vi "USRP_singlecarrierTDMUSRP1_conf.vi"() -> ()   [LabVIEW 2021]
uses:
  <vilib>/addons/Modulation/Analog/controls/Complex Data Waveform.ctl
  <vilib>/Analysis/coordinate.llb/Angle Units.ctl
  <vilib>/Analysis/coordinate.llb/Angle Range (Degree).ctl
  <vilib>/Analysis/coordinate.llb/Wrap Angle (scalar).vi
  system stop.vi
  <vilib>/measure/matone.llb/Extract Single Tone Information 1 Chan (CDB).vi
  <instrlib>/niUSRP/niUSRP Fetch Rx Data (CDB Cluster).vi
  <instrlib>/niUSRP/niUSRP Write Tx Data (CDB Cluster).vi
  <vilib>/addons/Modulation/niAMT.lvlib
  <vilib>/measure/NI_MAPro.lvlib
  <vilib>/Analysis/NI_AAL_Angle.lvlib
panel:
  in  "Tab Control":T1(tab)
  in  "IQ rate Tx":dbl=400000.0 format="%#_6p"
  in  "Tx Gain":dbl format="%#_6f"
  in  "Tx IP":refnum<k15>="192.168.10.2"
  out "coerced IQ rate Tx":dbl=100000.0 format="%#_6p"
  out "coerced carrier frequency Tx":dbl=100000.0 format="%#_6p"
  in  "Rx IP":refnum<k15>="192.168.10.2"
  in  "Rx gain":dbl format="%#_6f"
  in  "Frequency":dbl=10000.0 format="%#_13g"
  in  "Duration":dbl=0.01 format="%#_13g"
  out "coerced IQ rate Rx":dbl=100000.0 format="%#_6p"
  out "coerced carrier frequency Rx":dbl=100000.0 format="%#_6p"
  in  "number of samples":i64=4000
  in  "carrier frequency":dbl=2400000000.0 format="%#_6p"
  in  "Phase in deg":dbl
  out "Counter":dbl
  out "Waveform Graph":dbl[](graph)
  out "Boolean":bool
  out "detected frequency":dbl format="%.2p"
  out "detected Amplitude":dbl format="%.2p"
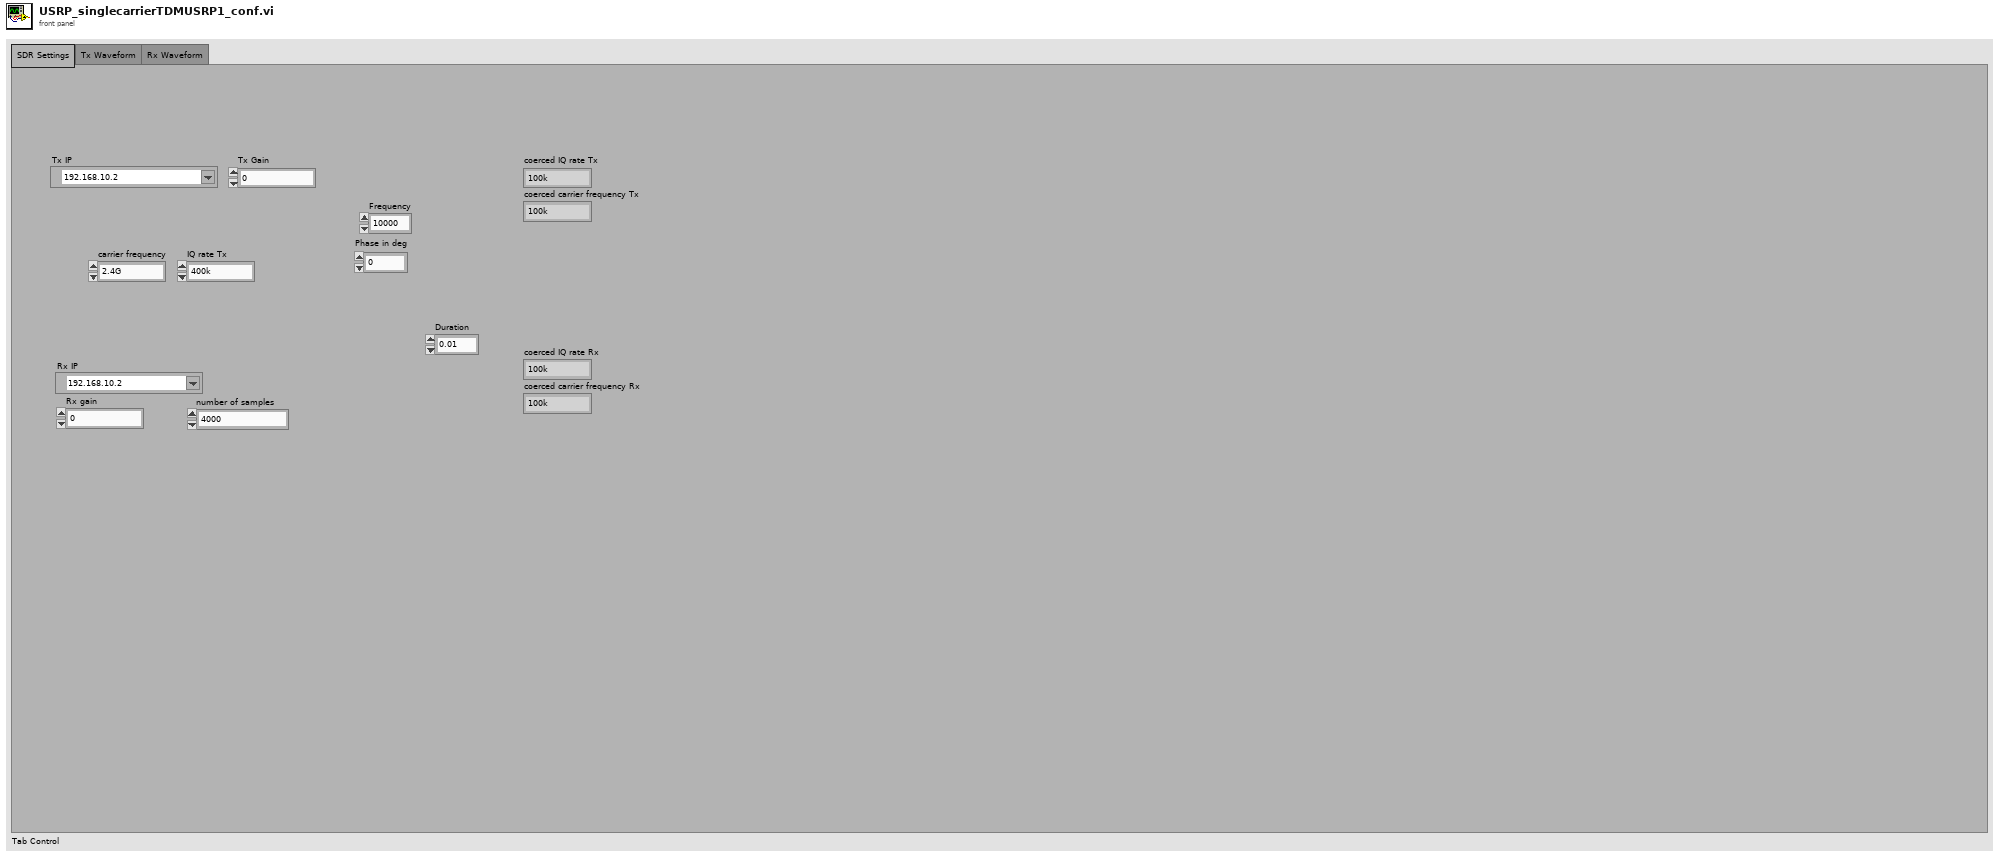
[diagram p1: front panel]
types:
  T1 = enum32{"SDR Settings", "Tx Waveform", "Rx Waveform"}
  T2 = typedef "niAMT.lvlib/Complex Data Waveform.ctl" = cluster{"t0":dbl, "dt":dbl, "Y":cdb[]}
  T3 = typedef "NI_AAL_Angle.lvlib/Angle Range (Degree).ctl" = u16
  T4 = typedef "NI_AAL_Angle.lvlib/Angle Units.ctl" = i32
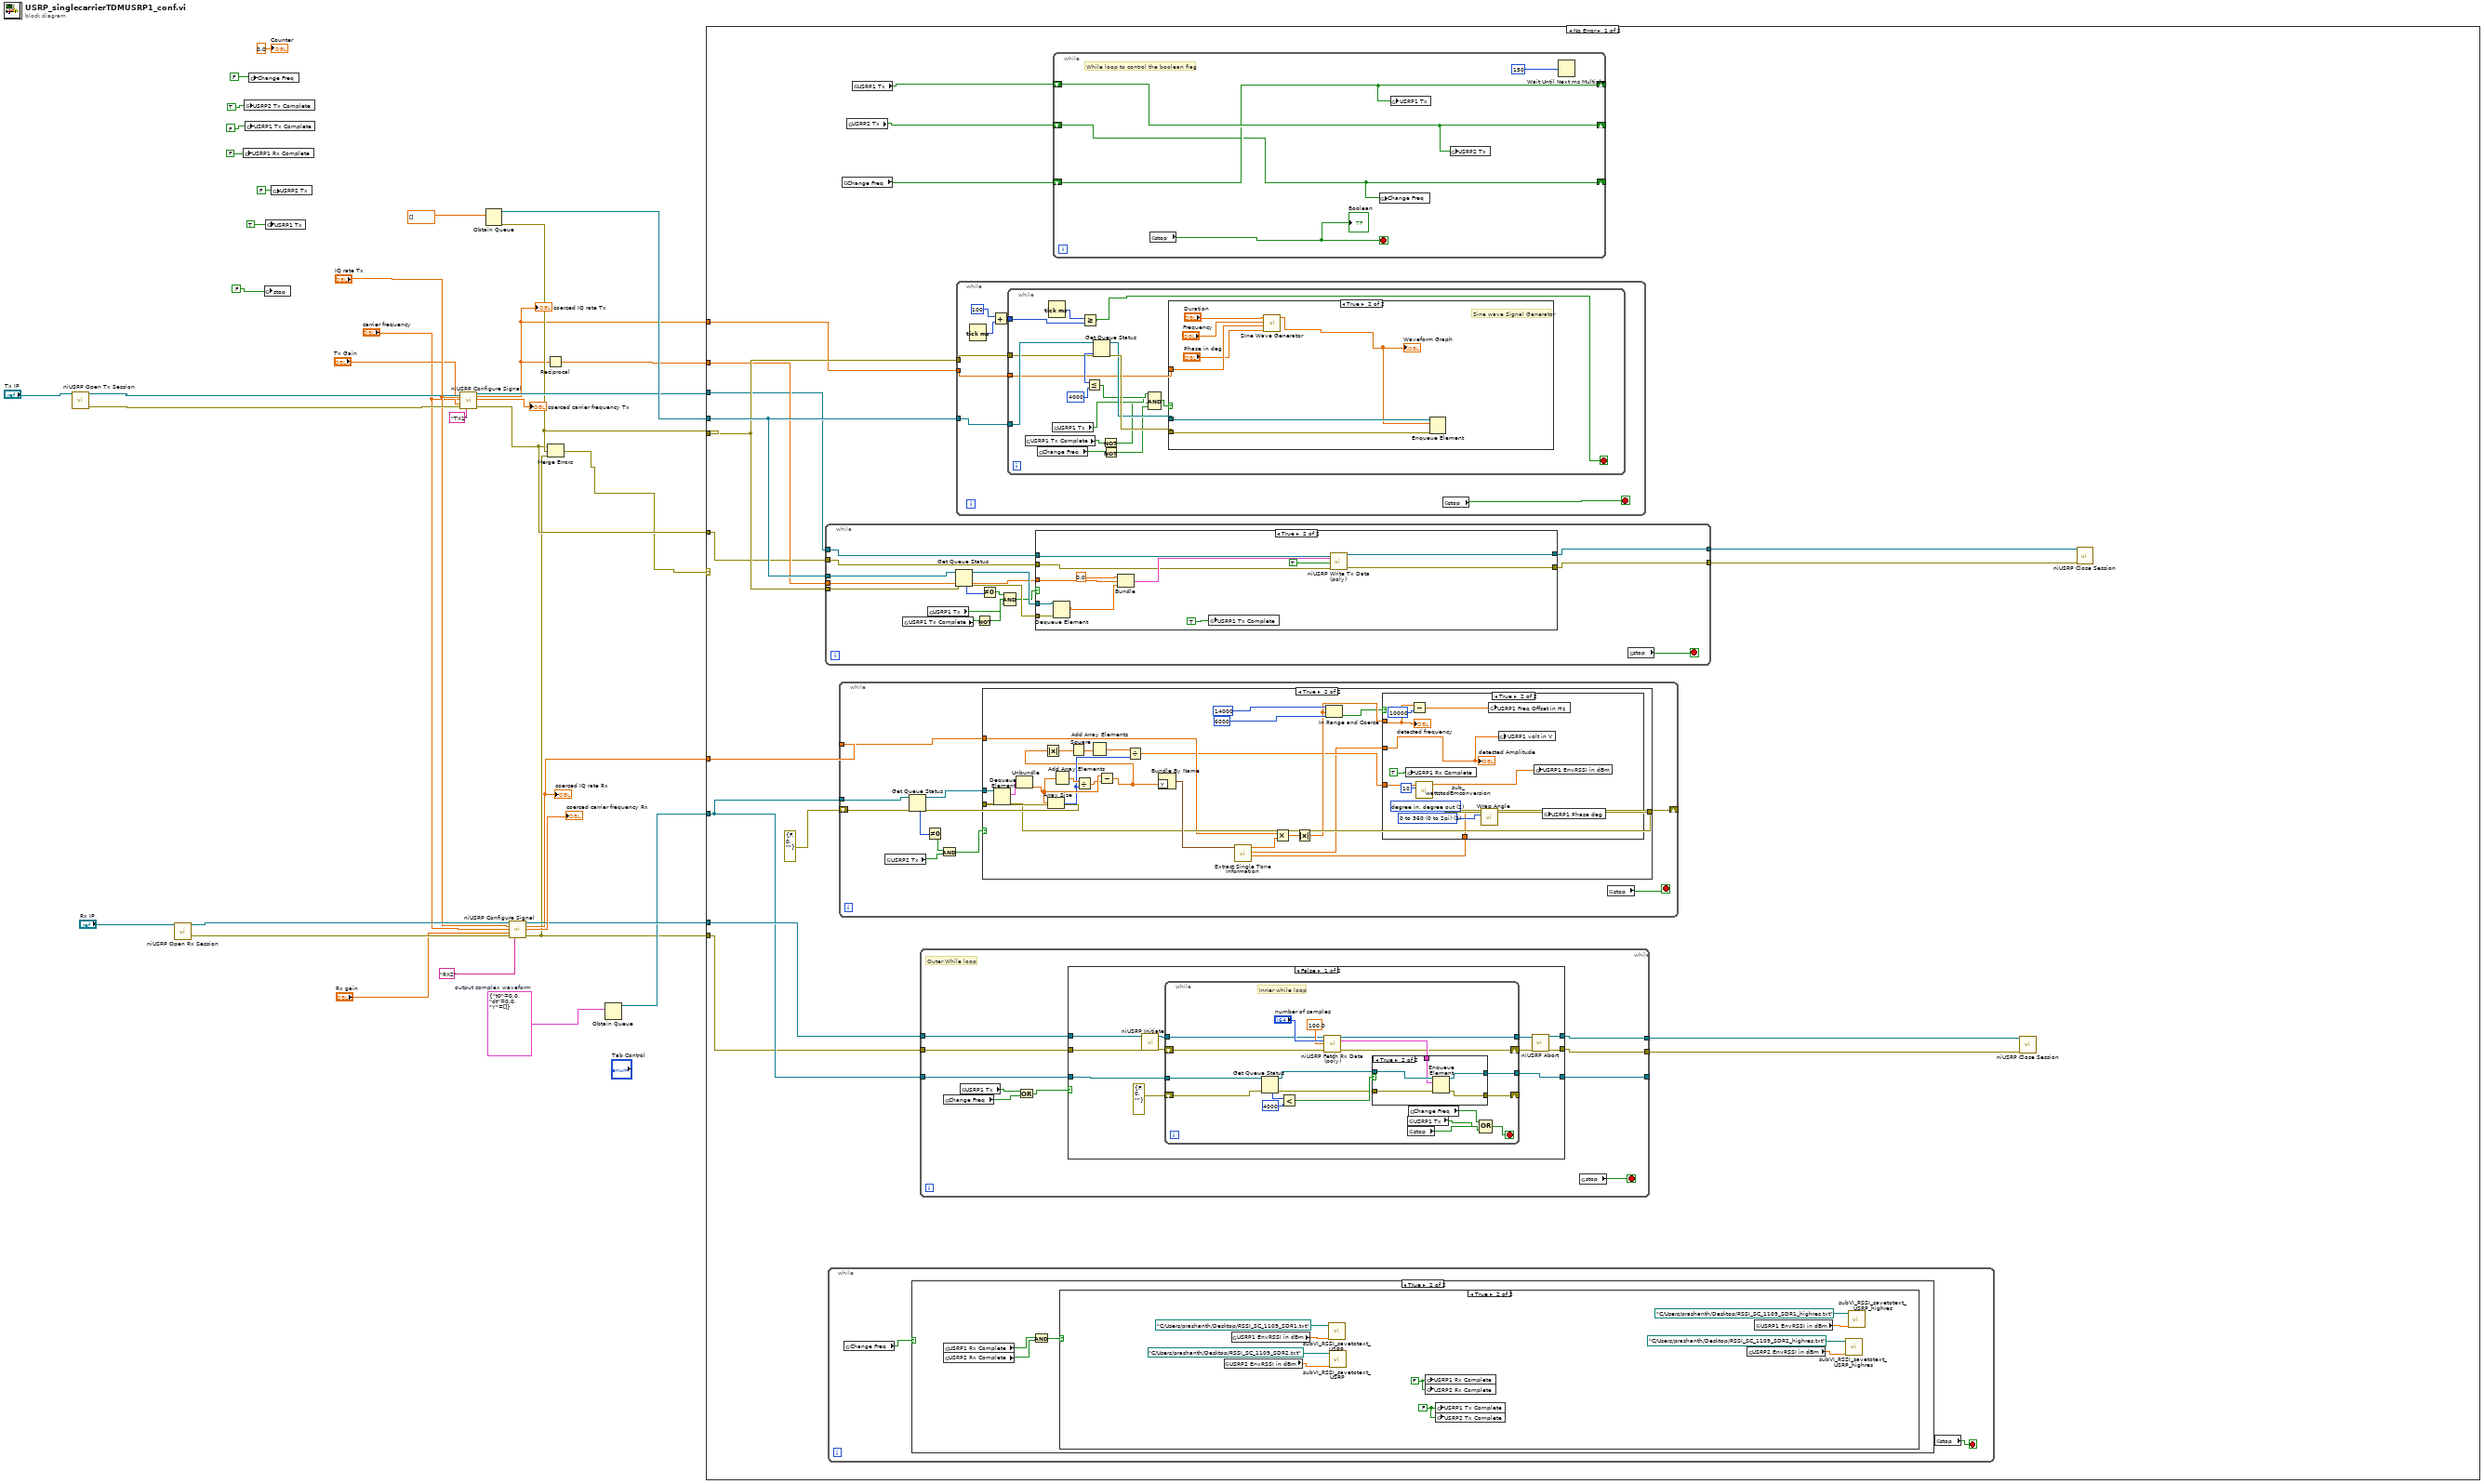
[diagram p0: block diagram]
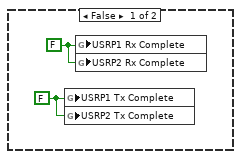
[diagram p3: hidden frame]
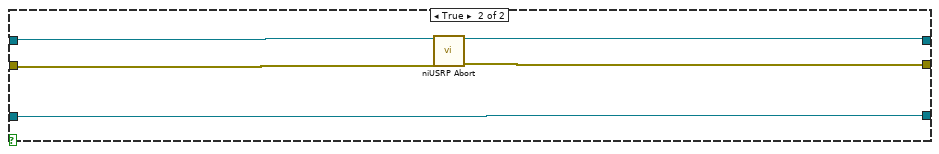
[diagram p6: hidden frame]
diagram:
  w9 = T2 {"t0"=0.0, "dt"=0.0, "Y"=[]}  # output complex waveform
  n1 = call <instrlib>:"niUSRP Open Tx Session.vi"("device names"="Tx IP") -> ("session handle out"=w34:refnum<k15>, "error out"=w33:errorcluster)  [unwired: 13 in]
  n2 = call <instrlib>:"niUSRP Open Rx Session.vi"("device names"="Rx IP") -> ("session handle out"=w31:refnum<k15>, "error out"=w30:errorcluster)  [unwired: 13 in]
  n3 = global write "system stop.vi" "USRP1 Rx Complete"(FALSE) -> ()
  n4 = global write "system stop.vi" "USRP2 Tx Complete"(TRUE) -> ()
  n5 = global write "system stop.vi" "USRP1 Tx Complete"(FALSE) -> ()
  n6 = global write "system stop.vi" "Change Freq"(FALSE) -> ()
  n7 = global write "system stop.vi" "stop"(FALSE) -> ()
  n8 = global write "system stop.vi" "USRP1 Tx"(TRUE) -> ()
  n9 = global write "system stop.vi" "USRP2 Tx"(FALSE) -> ()
  n10 = call <instrlib>:"niUSRP Configure Signal.vi"("session handle"=w34, "IQ rate"="IQ rate Tx", "carrier frequency"="carrier frequency", "gain"="Tx Gain", "error in (no error)"=w33, "active antenna"="TX1") -> ("session handle out"=w16:refnum<k15>, "coerced IQ rate"=w13:dbl, "coerced carrier frequency"=→"coerced carrier frequency Tx":dbl, "error out"=w12:errorcluster)  [unwired: 5 in, 1 out]
  "coerced IQ rate Tx" <- w13
  n11 = Obtain Queue(element data type=dbl[] []) -> (queue out=w17:refnum<queue>, error out=w14:errorcluster)  [unwired: 4 in, 1 out]
  n12 = call <instrlib>:"niUSRP Configure Signal.vi"("session handle"=w31, "IQ rate"="IQ rate Tx", "carrier frequency"="carrier frequency", "gain"="Rx gain", "error in (no error)"=w30, "active antenna"="RX2") -> ("session handle out"=w10:refnum<k15>, "coerced IQ rate"=w7:dbl, "coerced carrier frequency"=→"coerced carrier frequency Rx":dbl, "error out"=w6:errorcluster)  [unwired: 5 in, 1 out]
  "coerced IQ rate Rx" <- w7
  n13 = Reciprocal(x=w13) -> (1/x=w15:dbl)
  n14 = Merge Errors(w12, w14, w6) -> (w4:errorcluster)
  n15 = Obtain Queue(element data type=w9) -> (queue out=w8:refnum<queue>)  [unwired: 4 in, 2 out]
  n16 = case shown="No Error" w4 {
    tunnel: w14 -> [w52 _]
    tunnel: w17 -> [w53 _]
    tunnel: w16 -> [w50 _]
    tunnel: w15 -> [w51 _]
    tunnel: w13 -> [w49 _]
    tunnel: w12 -> [w48 _]
    tunnel: w10 -> [w46 _]
    tunnel: w8 -> [w45 _]
    tunnel: w7 -> [w44 _]
    tunnel: w6 -> [w43 _]
    frame No Error {
      n17 = while {
        tunnel: w52 -> [w219]
        tunnel: w51 -> [w218]
        tunnel: w50 -> [w215]
        tunnel: w48 -> [w214]
        tunnel: [w210] -> w39
        tunnel: [w209] -> w38
        tunnel: w53 -> [w222]
        stop <- w216 stop-if-true
        n18 = global read "system stop.vi" "USRP1 Tx Complete"() -> (w211:bool)
        n19 = global read "system stop.vi" "USRP1 Tx"() -> (w207:bool)
        n20 = Get Queue Status(queue=w222, error in (no error)=w219) -> (queue out=w221:refnum<queue>, error out=w220:errorcluster, # elements in queue=w217:i32)  [unwired: 1 in, 5 out]
        n21 = Not(x=w211) -> (.not. x?=w212:bool)
        n22 = Not Equal To 0?(x=w217) -> (x != 0?=w213:bool)
        n23 = Compound Arithmetic op=AND(w213, w212, w207) -> (w208:bool)
        n24 = case shown="True" w208 {
          tunnel: w221 -> [_ w236]
          tunnel: w220 -> [_ w235]
          tunnel: w218 -> [_ w234]
          tunnel: w215 -> [w224 w227]
          tunnel: w214 -> [w223 w226]
          tunnel: [w224 w230] -> w210
          tunnel: [w223 w228] -> w209
          frame False {
          }
          frame True {
            n25 = Dequeue Element(queue=w236, error in (no error)=w235) -> (element=w225:dbl[])  [unwired: 1 in, 3 out]
            n26 = Bundle(0.0, w234, w225) -> (w233:cluster{dbl, dbl, dbl[]})  [unwired: 1 in]
            n27 = global write "system stop.vi" "USRP1 Tx Complete"(TRUE) -> ()
            n28 = call-poly <instrlib>:"niUSRP Write Tx Data (poly).vi"("session handle"=w227, "data"=w233, "end of data?"=TRUE, "error in (no error)"=w226) -> ("session handle out"=w230:refnum<k15>, "error out"=w228:errorcluster)  [unwired: 10 in]
          }
        }
        n29 = global read "system stop.vi" "stop"() -> (w216:bool)
      }
      n30 = while {
        stop <- w54 stop-if-true
        n31 = global read "system stop.vi" "Change Freq"() -> (w55:bool)
        n32 = case shown="True" w55 {
          frame False {
          }
          frame True {
            n33 = global read "system stop.vi" "USRP1 Rx Complete"() -> (w58:bool)
            n34 = global read "system stop.vi" "USRP2 Rx Complete"() -> (w57:bool)
            n35 = And(x=w58, y=w57) -> (x .and. y?=w56:bool)
            n36 = case shown="True" w56 {
              frame False {
                w60 = FALSE
                w59 = FALSE
                n37 = global write "system stop.vi" "USRP1 Tx Complete"(w60) -> ()
                n38 = global write "system stop.vi" "USRP2 Tx Complete"(w60) -> ()
                n39 = global write "system stop.vi" "USRP1 Rx Complete"(w59) -> ()
                n40 = global write "system stop.vi" "USRP2 Rx Complete"(w59) -> ()
              }
              frame True {
                w70 = FALSE
                w69 = FALSE
                n41 = global read "system stop.vi" "USRP2 EnvRSSI in dBm"() -> (w61:dbl)
                n42 = global read "system stop.vi" "USRP1 EnvRSSI in dBm"() -> (w63:dbl)
                n43 = call "subVI_RSSI_savetotext_USRP.vi"("RSSI"=w63, "file path (dialog if empty)"=path "C:/Users/prashanth/Desktop/RSSI_SC_1109_SDR1.txt") -> ()  [unwired: 10 in]
                n44 = call "subVI_RSSI_savetotext_USRP.vi"("RSSI"=w61, "file path (dialog if empty)"=path "C:/Users/prashanth/Desktop/RSSI_SC_1109_SDR2.txt") -> ()  [unwired: 10 in]
                n45 = global write "system stop.vi" "USRP1 Rx Complete"(w69) -> ()
                n46 = global write "system stop.vi" "USRP2 Rx Complete"(w69) -> ()
                n47 = global write "system stop.vi" "USRP1 Tx Complete"(w70) -> ()
                n48 = global write "system stop.vi" "USRP2 Tx Complete"(w70) -> ()
                n49 = global read "system stop.vi" "USRP2 EnvRSSI in dBm"() -> (w67:dbl)
                n50 = global read "system stop.vi" "USRP1 EnvRSSI in dBm"() -> (w65:dbl)
                n51 = call "subVI_RSSI_savetotext_USRP_highres.vi"("RSSI"=w67, "file path (dialog if empty)"=path "C:/Users/prashanth/Desktop/RSSI_SC_1109_SDR2_highres.txt") -> ()  [unwired: 10 in]
                n52 = call "subVI_RSSI_savetotext_USRP_highres.vi"("RSSI"=w65, "file path (dialog if empty)"=path "C:/Users/prashanth/Desktop/RSSI_SC_1109_SDR1_highres.txt") -> ()  [unwired: 10 in]
              }
            }
          }
        }
        n53 = global read "system stop.vi" "stop"() -> (w54:bool)
      }
      n54 = while {
        tunnel: w45 -> [w167]
        shift-right: [w165] -> _
        shift-left: errorcluster {"status"=FALSE, "code"=0, "source"=""} ("error in (no error)") -> [w166]
        tunnel: w44 -> [w164]
        stop <- w163 stop-if-true
        n55 = global read "system stop.vi" "USRP2 Tx"() -> (w162:bool)
        n56 = Get Queue Status(queue=w167, error in (no error)=w166) -> (queue out=w169:refnum<queue>, error out=w168:errorcluster, # elements in queue=w170:i32)  [unwired: 1 in, 5 out]
        n57 = Not Equal To 0?(x=w170) -> (x != 0?=w161:bool)
        n58 = And(x=w161, y=w162) -> (x .and. y?=w160:bool)
        n59 = case shown="True" w160 {
          tunnel: w169 -> [_ w194]
          tunnel: w168 -> [w171 w193]
          tunnel: [w171 w187] -> w165
          tunnel: w164 -> [_ w185]
          frame False {
          }
          frame True {
            n60 = Dequeue Element(queue=w194, error in (no error)=w193) -> (element=w192:T2, error out=w187:errorcluster)  [unwired: 1 in, 2 out]
            n61 = Unbundle(w192) -> ("Y"=w182:cdb[])  [unwired: 2 out]
            n62 = Array Size(array=w182) -> (size(s)=w179:i32)
            n63 = Add Array Elements(numeric array=w182) -> (sum=w191:cdb)
            n64 = Divide(x=w191, y=w179) -> (x/y=w180:cdb)
            n65 = Subtract(x=w182, y=w180) -> (x-y=w174:cdb[])
            n66 = Absolute Value(x=w174) -> (abs(x)=w181:dbl[])
            n67 = Square(x=w181) -> (x^2=w178:dbl[])
            n68 = Add Array Elements(numeric array=w178) -> (sum=w177:dbl)
            n69 = Divide(x=w177, y=w179) -> (x/y=w176:dbl)
            n70 = Bundle By Name("Y"=w174) -> (w188:waveform(cdb))  [unwired: 1 in]
            n71 = call-poly <vilib>:"Extract Single Tone Information.vi"("time signal in"=w188) -> ("detected phase (deg)"=w175:dbl, "detected amplitude"=w173:dbl, "detected frequency"=w186:dbl)  [unwired: 5 in, 3 out]
            n72 = Multiply(x=w185, y=w186) -> (x*y=w184:dbl)
            n73 = Absolute Value(x=w184) -> (abs(x)=w183:dbl)
            n74 = In Range and Coerce(upper limit=14000, x=w183, lower limit=6000) -> (In Range?=w172:bool)  [unwired: 1 out]
            n75 = case shown="True" w172 {
              tunnel: w183 -> [_ w205]
              tunnel: w173 -> [_ w195]
              tunnel: w176 -> [_ w202]
              tunnel: w175 -> [_ w197]
              frame False {
              }
              frame True {
                w199 = T3 2 items=["none", "-180 to 180 (-pi to pi)", "0 to 360 (0 to 2pi)"] ("angle range")
                w200 = T4 2 items=["radian in, radian out", "radian in, degree out", "degree in, degree out", "degree in, radian out"] ("angle units")
                n76 = global write "system stop.vi" "USRP1 Rx Complete"(TRUE) -> ()
                n77 = Subtract(x=w205, y=10000) -> (x-y=w203:dbl)
                n78 = call "sub_wattstodBmconversion.vi"("Amp or Power"=10, "detected amplitude"=w202) -> ("Numeric"=w201:dbl)  [unwired: 9 in]
                n79 = call-poly <vilib>:"Wrap Angle.vi"("angle units"=w200, "angle range"=w199, "angle in"=w197) -> ("angle out"=w198:dbl)  [unwired: 7 in, 1 out]
                n80 = global write "system stop.vi" "USRP1 Freq Offset in Hz"(w203) -> ()
                n81 = global write "system stop.vi" "USRP1 volt in V"(w195) -> ()
                n82 = global write "system stop.vi" "USRP1 EnvRSSI in dBm"(w201) -> ()
                n83 = global write "system stop.vi" "USRP1 Phase deg"(w198) -> ()
                "detected frequency" <- w205
                "detected Amplitude" <- w195
              }
            }
          }
        }
        n84 = global read "system stop.vi" "stop"() -> (w163:bool)
      }
      n85 = global read "system stop.vi" "Change Freq"() -> (w41:bool)
      n86 = global read "system stop.vi" "USRP2 Tx"() -> (w40:bool)
      n87 = global read "system stop.vi" "USRP1 Tx"() -> (w42:bool)
      n88 = while {
        tunnel: w46 -> [w114]
        tunnel: w43 -> [w113]
        tunnel: [w108] -> w37
        tunnel: [w107] -> w36
        tunnel: w45 -> [w116]
        tunnel: [w112] -> _
        stop <- w115 stop-if-true
        # "Outer While loop"
        n89 = global read "system stop.vi" "Change Freq"() -> (w109:bool)
        n90 = global read "system stop.vi" "USRP1 Tx"() -> (w110:bool)
        n91 = Compound Arithmetic op=OR(w110, w109) -> (w111:bool)
        n92 = case shown="False" w111 {
          tunnel: w114 -> [w119 w159]
          tunnel: w116 -> [w127 w155]
          tunnel: w113 -> [w118 w157]
          tunnel: [w122 w158] -> w108
          tunnel: [w121 w156] -> w107
          tunnel: [w117 w155] -> w112
          frame False {
            n93 = call <instrlib>:"niUSRP Initiate.vi"("session handle"=w119, "error in (no error)"=w118) -> ("session handle out"=w125:refnum<k15>, "error out"=w124:errorcluster)  [unwired: 12 in]
            n94 = while {
              tunnel: w127 -> [w147]
              shift-right: [w131] -> w120
              shift-left: w124 -> [w133]
              shift-right: [w146] -> _
              shift-left: errorcluster {"status"=FALSE, "code"=0, "source"=""} ("error in (no error)") -> [w145]
              tunnel: w125 -> [w134]
              tunnel: [w132] -> w123
              tunnel: [w128] -> w117
              stop <- w137 stop-if-true
              # "Inner while loop"
              n95 = Get Queue Status(queue=w147, error in (no error)=w145) -> (queue out=w140:refnum<queue>, error out=w141:errorcluster, # elements in queue=w144:i32)  [unwired: 1 in, 5 out]
              n96 = Less?(x=w144, y=4000) -> (x < y?=w142:bool)
              n97 = call-poly <instrlib>:"niUSRP Fetch Rx Data (poly).vi"("session handle"=w134, "number of samples"="number of samples", "timeout"=100.0, "error in (no error)"=w133) -> ("session handle out"=w132:refnum<k15>, "data"=w138:cluster{"t0":dbl, "dt":dbl, "Y":cdb[]}, "error out"=w131:errorcluster)  [unwired: 8 in, 1 out]
              n98 = case shown="True" w142 {
                tunnel: w141 -> [w149 w154]
                tunnel: w140 -> [w148 w153]
                tunnel: w138 -> [_ w152]
                tunnel: [w149 w151] -> w146
                tunnel: [w148 w150] -> w128
                frame False {
                }
                frame True {
                  n99 = Enqueue Element(queue=w153, element=w152, error in (no error)=w154) -> (queue out=w150:refnum<queue>, error out=w151:errorcluster)  [unwired: 1 in, 1 out]
                }
              }
              n100 = global read "system stop.vi" "USRP1 Tx"() -> (w130:bool)
              n101 = global read "system stop.vi" "stop"() -> (w136:bool)
              n102 = global read "system stop.vi" "Change Freq"() -> (w129:bool)
              n103 = Compound Arithmetic op=OR(w129, w130, w136) -> (w137:bool)
            }
            n104 = call <instrlib>:"niUSRP Abort.vi"("session handle"=w123, "error in (no error)"=w120) -> ("session handle out"=w122:refnum<k15>, "error out"=w121:errorcluster)  [unwired: 12 in]
          }
          frame True {
            n105 = call <instrlib>:"niUSRP Abort.vi"("session handle"=w159, "error in (no error)"=w157) -> ("session handle out"=w158:refnum<k15>, "error out"=w156:errorcluster)  [unwired: 12 in]
          }
        }
        n106 = global read "system stop.vi" "stop"() -> (w115:bool)
      }
      n107 = while {
        tunnel: w52 -> [w81]
        tunnel: w49 -> [w80]
        tunnel: w53 -> [w82]
        stop <- w76 stop-if-true
        n108 = Tick Count (ms)() -> (millisecond timer value=w78:u32)
        n109 = Add(x=100, y=w78) -> (x+y=w77:u32)
        n110 = while {
          tunnel: w81 -> [w94]
          tunnel: w80 -> [w93]
          tunnel: w77 -> [w88]
          tunnel: w82 -> [w95]
          stop <- w84 stop-if-true
          n111 = global read "system stop.vi" "USRP1 Tx Complete"() -> (w86:bool)
          n112 = global read "system stop.vi" "Change Freq"() -> (w85:bool)
          n113 = Tick Count (ms)() -> (millisecond timer value=w89:u32)
          n114 = global read "system stop.vi" "USRP1 Tx"() -> (w91:bool)
          n115 = Greater Or Equal?(x=w89, y=w88) -> (x >= y?=w84:bool)
          n116 = Get Queue Status(queue=w95, error in (no error)=w94) -> (queue out=w96:refnum<queue>, error out=w97:errorcluster, # elements in queue=w99:i32)  [unwired: 1 in, 5 out]
          n117 = Less Or Equal?(x=w99, y=4000) -> (x <= y?=w92:bool)
          n118 = Not(x=w86) -> (.not. x?=w87:bool)
          n119 = Not(x=w85) -> (.not. x?=w83:bool)
          n120 = Compound Arithmetic op=AND(w92, w91, w87, w83) -> (w90:bool)
          n121 = case shown="True" w90 {
            tunnel: w97 -> [_ w106]
            tunnel: w96 -> [_ w105]
            tunnel: w93 -> [_ w102]
            frame False {
            }
            frame True {
              # "Sine wave Signal Generator"
              n122 = call "SIne Wave Generator.vi"("Phase in deg"="Phase in deg", "Sampling rate"=w102, "Frequency"="Frequency", "Duration"="Duration") -> ("Array"=w100:dbl[])  [unwired: 6 in, 1 out]
              "Waveform Graph" <- w100
              n123 = Enqueue Element(queue=w105, element=w100, error in (no error)=w106) -> ()  [unwired: 1 in, 3 out]
            }
          }
        }
        n124 = global read "system stop.vi" "stop"() -> (w76:bool)
      }
      n125 = while {
        shift-right: [w73] -> _
        shift-left: w42 -> [w75]
        shift-right: [w75] -> _
        shift-left: w40 -> [w72]
        shift-right: [w72] -> _
        shift-left: w41 -> [w73]
        stop <- w74 stop-if-true
        # "While loop to control the boolean flag"
        n126 = global read "system stop.vi" "stop"() -> (w74:bool)
        "Boolean" <- w74
        n127 = global write "system stop.vi" "Change Freq"(w72) -> ()
        n128 = global write "system stop.vi" "USRP1 Tx"(w73) -> ()
        n129 = global write "system stop.vi" "USRP2 Tx"(w75) -> ()
        n130 = Wait Until Next ms Multiple(millisecond multiple=150) -> ()  [unwired: 1 out]
      }
      n131 = call <instrlib>:"niUSRP Close Session.vi"("session handle"=w37, "error in (no error)"=w36) -> ()  [unwired: 13 in, 1 out]
      n132 = call <instrlib>:"niUSRP Close Session.vi"("session handle"=w39, "error in (no error)"=w38) -> ()  [unwired: 13 in, 1 out]
    }
    frame Error {
    }
  }
  "Counter" <- 0.0 ("Counter")
